vi "read_kml.vi"(8 "error in":errorcluster, 10 "XPath Expression":string="/kml/Document/Folder/Placemark/LineString/coordinates", 11 "KML File Path":path) -> (0 "error out":errorcluster, 3 "array(lon, lat)":dbl[][](array[numeric]))   [LabVIEW 2020]
uses:
  <vilib>/xml/Close Reference(Node).vi
  <vilib>/xml/NI_XML.lvlib
  <resource>/objmgr/DOMUserDefRef.rc
panel:
  out "size(s)":i32
  out "XML":string
  # "/kml/Document/Folder/Placemark/LineString/coordinates"
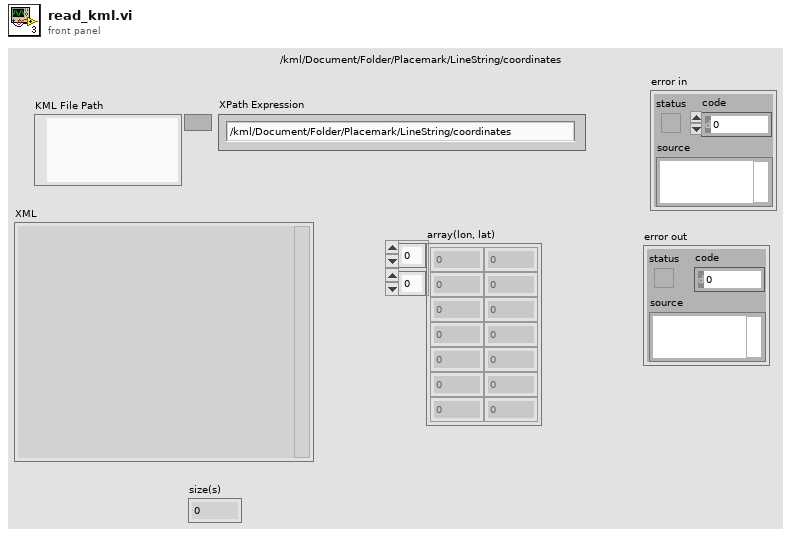
[diagram p1: front panel]
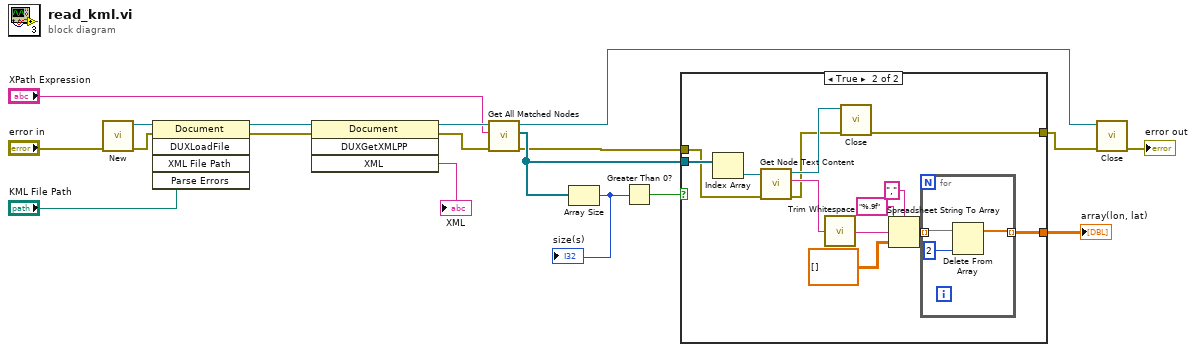
[diagram p0: block diagram]
diagram:
  n1 = call <vilib>:"New.vi"("error in (no error)"="error in") -> ("error out"=w14:errorcluster, "DOM document out"=w18:refnum<k20>)  [unwired: 7 in]
  n2 = invoke class="Document" method="DUXLoadFile"(reference=w18, error in=w14, "XML File Path"="KML File Path") -> (reference out=w16:refnum<k20>, error out=w15:errorcluster)  [unwired: 2 in, 3 out]
  n3 = invoke class="Document" method="DUXGetXMLPP"(reference=w16, error in=w15) -> (reference out=w12:refnum<k20>, error out=w10:errorcluster, "XML"=→"XML":string)  [unwired: 2 in, 1 out]
  n4 = call <vilib>:"Get All Matched Nodes.vi"("error in (no error)"=w10, "XPath expression"="XPath Expression", "node in"=w12) -> ("error out"=w6:errorcluster, "node result array"=w7:refnum<k20>[], "node out"=w3:refnum<k20>)  [unwired: 6 in]
  n5 = Array Size(array=w7) -> (size(s)=w9:i32)
  "size(s)" <- w9
  n6 = Greater Than 0?(x=w9) -> (x > 0?=w8:bool)
  n7 = case shown="True" w8 {
    tunnel: w7 -> [_ w32]
    tunnel: w6 -> [w19 w23]
    tunnel: [_ w21] -> w5
    tunnel: [w19 w20] -> w4
    frame False {
    }
    frame True {
      n8 = Index Array(array=w32) -> (element=w31:refnum<k20>)  [unwired: 1 in]
      n9 = call <vilib>:"Get Node Text Content.vi"("error in (no error)"=w23, "node in"=w31) -> ("error out"=w22:errorcluster, "node text"=w26:string, "node out"=w30:refnum<k20>)  [unwired: 7 in]
      n10 = call <vilib>:"Trim Whitespace.vi"("string"=w26) -> ("trimmed string"=w25:string)  [unwired: 1 in]
      n11 = call-poly <vilib>:"Close.vi"("error in (no error)"=w22, "node"=w30) -> ("error out"=w20:errorcluster)  [unwired: 7 in]
      n12 = Spreadsheet String To Array(delimiter (Tab)=",", format string="%.9f", spreadsheet string=w25, array type (2D Dbl)=dbl[][] []) -> (array=w24:dbl[][])
      n13 = for {
        tunnel: w24 -> [w35] mode=indexing
        tunnel: [w33] -> w21 mode=indexing
        n14 = Delete From Array(array=w35, index=2) -> (array with subset deleted=w33:dbl[])  [unwired: 1 in, 1 out]
      }
    }
  }
  "array(lon, lat)" <- w5
  n15 = call-poly <vilib>:"Close.vi"("error in (no error)"=w4, "node"=w3) -> ("error out"=→"error out":errorcluster)  [unwired: 7 in]
